vi "Power.vi"(6 "Timeout (ms)":i32=1000, 8 "error in (no error)":errorcluster, 10 "Enable Drive":bool, 11 "FHPP in":refnum<class "FHPP.lvclass">) -> (0 "error out":errorcluster, 2 "Timeout":bool, 3 "FHPP out":refnum<class "FHPP.lvclass">)   [LabVIEW 2022 SP3, in "FHPP.lvclass"]
doc: "Power on/off drive. Wait for setting commited or timeout."
uses:
  FHPP.lvclass
  FHPP.lvclass/FHPP.ctl
  <vilib>/GPower/Timing/GPTiming.lvlib
  <vilib>/GPower/Timing/Library/Remaining/Remaining_ms.vi
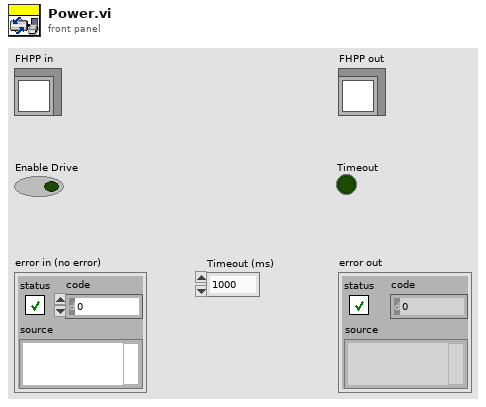
[diagram p1: front panel]
types:
  T1 = typedef "FHPP.lvclass/CCON.ctl" = cluster{"Enabled Drive":bool, "Stop":bool, "Open Brake":bool, "Reset Fault":bool, "Reserved":bool, "Lock Software Access":bool, "Operating Mode":T2}
  T2 = typedef "FHPP.lvclass/Operating Mode.ctl" = enum16{"Record Selection", "Direct Mode", "Reserved 1", "Reserved 2"}
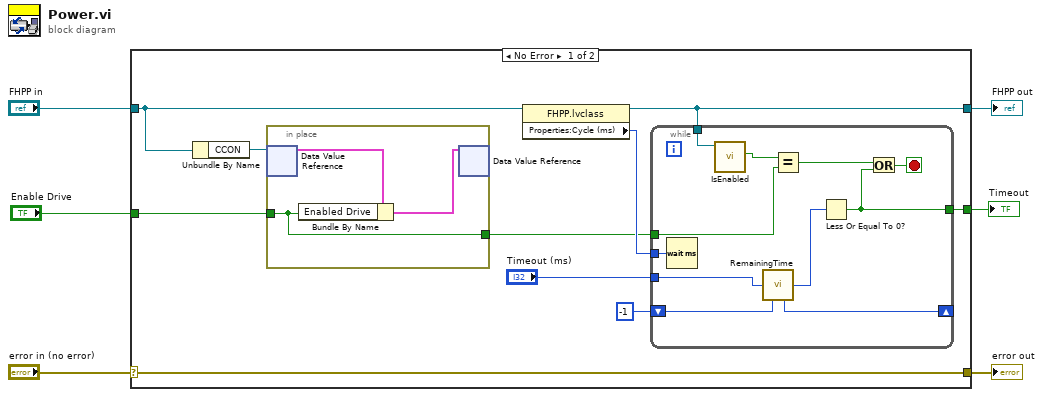
[diagram p0: block diagram]
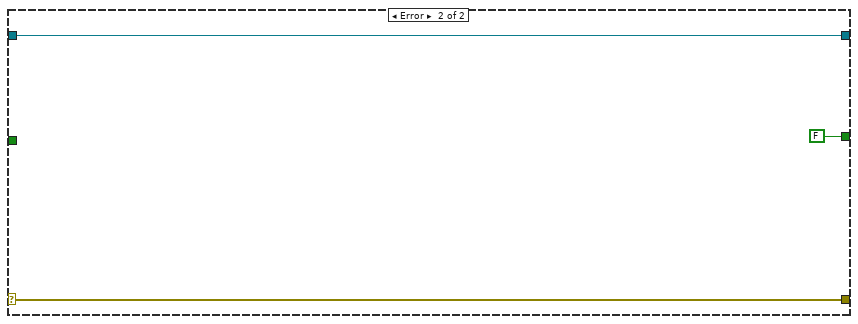
[diagram p2: hidden frame]
diagram:
  n1 = case shown="No Error" "error in (no error)" {
    selector: "error in (no error)" -> [w16 w33]
    tunnel: [w16 w33] -> w5
    tunnel: [w8 w32] -> w3
    tunnel: "FHPP in" -> [w10 w32]
    tunnel: "Enable Drive" -> [w14 _]
    tunnel: [w11 FALSE] -> w1
    frame No Error {
      n2 = Unbundle By Name(w10) -> ("CCON"=w15:refnum<data-value>)
      n3 = in-place {
        in-place-border: w14 -> [w28]
        in-place-border: [w28] -> w7
        n4 = in-place-dvr #1(w15) -> (w30:T1)  [unwired: 1 out]
        n5 = Bundle By Name(cluster=w30, "Enabled Drive"=w28) -> (w29:T1)
        n6 = in-place-dvr #1(w29) -> ()  [unwired: 2 out]
      }
      n7 = property class="FHPP.lvclass"(reference=w10) -> (reference out=w8:refnum<class "FHPP.lvclass">, "Properties:Cycle (ms)"=w9:i32)  [unwired: 1 in, 1 out]
      n8 = while {
        tunnel: "Timeout (ms)" -> [w27]
        shift-right: [w25] -> _
        shift-left: i64 -1 ("Start time out") -> [w26]
        tunnel: [w23] -> w11
        tunnel: w9 -> [w22]
        tunnel: w8 -> [w19]
        tunnel: w7 -> [w17]
        stop <- w21 stop-if-true
        n9 = Wait (ms)(milliseconds to wait=w22) -> ()  [unwired: 1 out]
        n10 = call-dynamic "IsEnabled.vi"("FHPP in"=w19) -> ("Drive Enabled"=w20:bool)  [unwired: 7 in, 3 out]
        n11 = call-poly <vilib>:"RemainingTime.vi"("Time period target"=w27, "Start time in"=w26) -> ("Remaining time"=w24:i32, "Start time out"=w25:i64)  [unwired: 9 in, 3 out]
        n12 = Equal?(x=w20, y=w17) -> (x = y?=w18:bool)
        n13 = Less Or Equal To 0?(x=w24) -> (x <= 0?=w23:bool)
        n14 = Or(x=w18, y=w23) -> (x .or. y?=w21:bool)
      }
    }
    frame Error {
    }
  }
  "error out" <- w5
  "FHPP out" <- w3
  "Timeout" <- w1
